vi "Connect.vi"(8 "error in (no error)":errorcluster, 11 "CameraDemo in":refnum<class "CameraDemo.lvclass">) -> (0 "error out":errorcluster, 3 "CameraDemo out":refnum<class "CameraDemo.lvclass">)   [LabVIEW 2020, in "CameraI2COUSB.lvlib" / "CameraDemo.lvclass"]
doc: "Open connection to camera"
uses:
  CameraDemo.lvclass
  CameraDemo.lvclass/CameraDemo.ctl
  I2CDriver/II2COUSB/II2COUSB/II2COUSB.lvclass
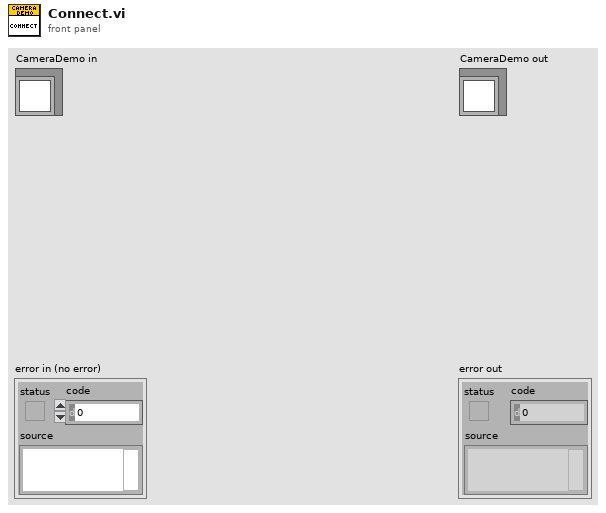
[diagram p1: front panel]
types:
  T1 = typedef "II2COUSB.lvlib/II2COUSB.lvclass/ConnectionParams.ctl" = cluster{"Vid":u16, "Pid":u16, "Device Index":u32, "u32_I2Cclk":u32}
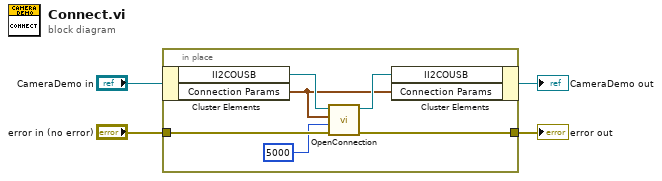
[diagram p0: block diagram]
diagram:
  n1 = in-place {
    in-place-border: "error in (no error)" -> [w10]
    in-place-border: [w9] -> w3
    n2 = in-place-cluster #1("CameraDemo in") -> ("II2COUSB"=w8:refnum<class "II2COUSB.lvclass">, "Connection Params"=w5:T1)
    n3 = call-dynamic "OpenConnection.vi"("error in (no error)"=w10, "Timeout (ms)"=u32 5000, "Connection Params"=w5, "II2COUSB in"=w8) -> ("error out"=w9:errorcluster, "II2COUSB out"=w7:refnum<class "II2COUSB.lvclass">)  [unwired: 6 in]
    n4 = in-place-cluster #1("II2COUSB"=w7, "Connection Params"=w5) -> (→"CameraDemo out":refnum<class "CameraDemo.lvclass">)
  }
  "error out" <- w3
